vi "act_hvr.vi"() -> (0 "HVR_4":bool, 1 "HVR_3":bool, 2 "HVR_2":bool, 3 "HVR_1":bool)   [LabVIEW 2018]
uses:
  <vilib>/rvi/DataTransferAndStorage/Container/Common/niFpgaContainerExecOnDevCompGetState.vi
  <vilib>/rvi/Emulation/niFpgaEmulationIsFPGAContextNoSignature.vi
  <vilib>/rvi/DataTransferAndStorage/Container/Common/niFpgaContainerGetUniqueNameForEmu.vi
  <vilib>/rvi/Memory/Memory_Emulation/niFpgaMemoryEmulationCacheClearOnFirstRun.vi
  <vilib>/rvi/Memory/Memory_Emulation/nirvimemoryEmulationManagerCache_MakeExclusive.vi
  <vilib>/rvi/Memory/Memory_Emulation/niFpgaMemoryEmulationValidateCache.vi
  <vilib>/rvi/Memory/Memory_Emulation/nirvimemoryEmulationManagerCache_InsertValue.vi
  <vilib>/Utility/error.llb/Clear Errors.vi
  <vilib>/rvi/Memory/Memory_Emulation/nirvimemoryEmulationManagerCache_ReleaseExclusive.vi
  <vilib>/rvi/Memory/Memory_Emulation/nirvimemoryEmulationManagerCache_GetValue.vi
  <vilib>/rvi/Memory/Memory_Emulation/nirvimemoryEmulationManagerCache_SetValue.vi
  <vilib>/rvi/Emulation/niFpgaProcessEmulError.vi
  <vilib>/rvi/Emulation/niFpgaSctlEmulationGetInTimedLoop.vi
  <vilib>/rvi/eio/common/nirviEmuTemplateMethod_errors.vi
  <vilib>/rvi/DataTransferAndStorage/Container/XNode/niFpgaContainer.xnode
  <vilib>/rvi/DataTransferAndStorage/Register/Emulation/niFpgaRegisterEmulationRefIn.vi
  <vilib>/eio/EIONode/EIONode.xnode
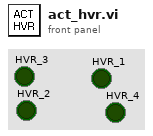
[diagram p1: front panel]
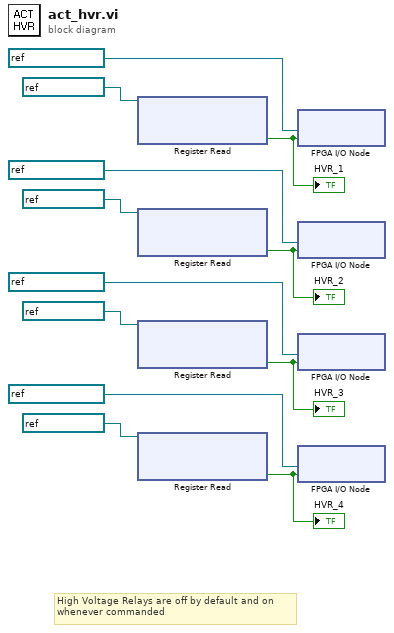
[diagram p0: block diagram]
diagram:
  # "High Voltage Relays are off by default and on\nwhenever commanded"
  n1 = xnode ("Register Read")("Register In"=refnum<k21> "REG_hvr_1") -> ("Data"=w4:bool)  [unwired: 1 out]
  "HVR_1" <- w4
  n2 = xnode ("Register Read")("Register In"=refnum<k21> "REG_hvr_2") -> ("Data"=w3:bool)  [unwired: 1 out]
  "HVR_2" <- w3
  n3 = xnode ("Register Read")("Register In"=refnum<k21> "REG_hvr_3") -> ("Data"=w2:bool)  [unwired: 1 out]
  "HVR_3" <- w2
  n4 = xnode ("Register Read")("Register In"=refnum<k21> "REG_hvr_4") -> ("Data"=w1:bool)  [unwired: 1 out]
  "HVR_4" <- w1
  n5 = xnode "FPGA I/O Node"("I/O Item"=w4, "FPGA I/O In"=refnum<k21> "Mod2/DIO12") -> ()  [unwired: 1 out]
  n6 = xnode "FPGA I/O Node"("I/O Item"=w3, "FPGA I/O In"=refnum<k21> "Mod2/DIO13") -> ()  [unwired: 1 out]
  n7 = xnode "FPGA I/O Node"("I/O Item"=w2, "FPGA I/O In"=refnum<k21> "Mod2/DIO14") -> ()  [unwired: 1 out]
  n8 = xnode "FPGA I/O Node"("I/O Item"=w1, "FPGA I/O In"=refnum<k21> "Mod2/DIO15") -> ()  [unwired: 1 out]
